vi "Set LibraryPaths to Include Icon Editor.vi"(8 "error in":errorcluster) -> (0 "error out":errorcluster, 2 "config modified?":bool)   [LabVIEW 2020]
doc: "Sets the LibraryPaths folder to point to the current project folder. This requires LabVIEW to restart to take affect."
uses:
  <vilib>/Utility/config.llb/NI_LVConfig.lvlib
  <vilib>/Utility/config.llb/Read Key (String).vi
  <vilib>/Utility/config.llb/Write Key (String).vi
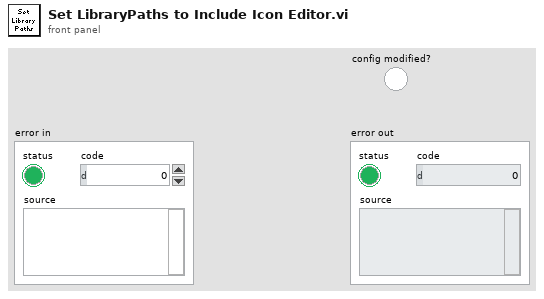
[diagram p1: front panel]
types:
  T1 = typedef "NI_LVConfig.lvlib/Config Data RefNum.ctl" = refnum<k1>
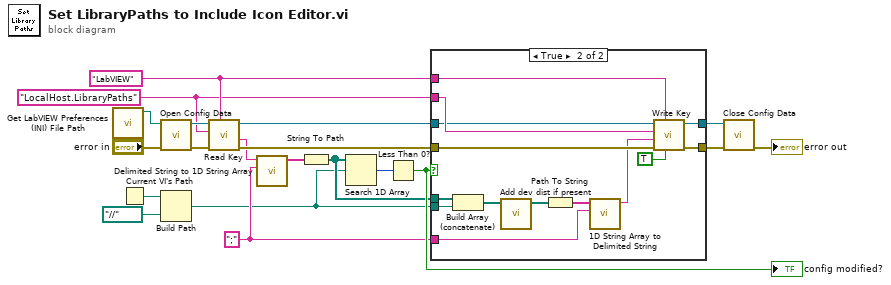
[diagram p0: block diagram]
diagram:
  w7 = ";" ("delimiter")
  w6 = "LabVIEW" ("section")
  w5 = "LocalHost.LibraryPaths" ("key")
  n1 = call <resource>:"Get LabVIEW Preferences (INI) File Path.vi"() -> ("LabVIEW Preferences (INI) File Path"=w2:path)  [unwired: 11 in]
  n2 = Current VI's Path() -> (path=w12:path)
  n3 = call <vilib>:"Open Config Data.vi"("error in (no error)"="error in", "configuration file path"=w2) -> ("error out"=w20:errorcluster, "refnum"=w14:T1)  [unwired: 7 in, 1 out]
  n4 = Build Path(base path=w12, name or relative path=path "../../..") -> (appended path=w1:path)
  n5 = call-poly <vilib>:"Read Key.vi"("section"=w6, "error in (no error)"=w20, "key"=w5, "refnum"=w14) -> ("error out"=w19:errorcluster, "value"=w11:string, "refnum out"=w4:T1)  [unwired: 4 in, 1 out]
  n6 = call <vilib>:"Delimited String to 1D String Array.vi"("delimiter"=w7, "delimited string"=w11) -> ("string array"=w10:string[])  [unwired: 9 in]
  n7 = String To Path(string=w10) -> (path=w8:path[])
  n8 = Search 1D Array(1D array=w8, element=w1) -> (index of element=w9:i32)  [unwired: 1 in]
  n9 = Less Than 0?(x=w9) -> (x < 0?=w15:bool)
  "config modified?" <- w15
  n10 = case shown="True" w15 {
    tunnel: w8 -> [_ w34]
    tunnel: w1 -> [_ w33]
    tunnel: w7 -> [_ w30]
    tunnel: w6 -> [_ w29]
    tunnel: w5 -> [_ w28]
    tunnel: w4 -> [w21 w26]
    tunnel: w19 -> [w22 w36]
    tunnel: [w21 w25] -> w3
    tunnel: [w22 w35] -> w18
    frame False {
    }
    frame True {
      n11 = Build Array (concatenate)(w34, w33) -> (w32:path[])
      n12 = call "Add dev dist if present.vi"("paths in"=w32) -> ("paths out"=w23:path[])  [unwired: 10 in]
      n13 = Path To String(path=w23) -> (string=w31:string[])
      n14 = call <vilib>:"1D String Array to Delimited String.vi"("delimiter"=w30, "string array"=w31) -> ("delimited string"=w27:string)  [unwired: 9 in]
      n15 = call-poly <vilib>:"Write Key.vi"("write raw string? (F)"=TRUE, "section"=w29, "error in (no error)"=w36, "value"=w27, "key"=w28, "refnum"=w26) -> ("error out"=w35:errorcluster, "refnum out"=w25:T1)  [unwired: 3 in, 1 out]
    }
  }
  n16 = call <vilib>:"Close Config Data.vi"("error in (no error)"=w18, "refnum"=w3) -> ("error out"=→"error out":errorcluster)  [unwired: 8 in, 1 out]
